vi "Serial Port Receive.vi"(8 "error in (no error)":errorcluster, 11 "Port handle in":refnum<k24>) -> (0 "error out":errorcluster, 2 "Message":u8[](array[numeric]) format="%.0x", 3 "Port handle out":refnum<k24>)   [LabVIEW 2015, in "VC940.lvlib"]
uses:
  VC940.lvlib
panel:
  out "Iteration":i32
  out "Message interval/ms":u32
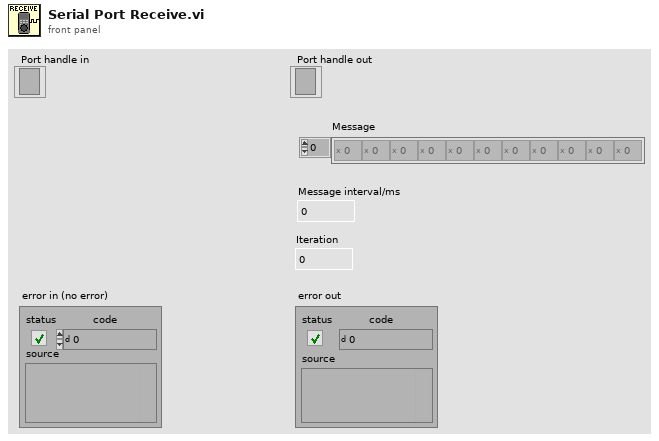
[diagram p1: front panel]
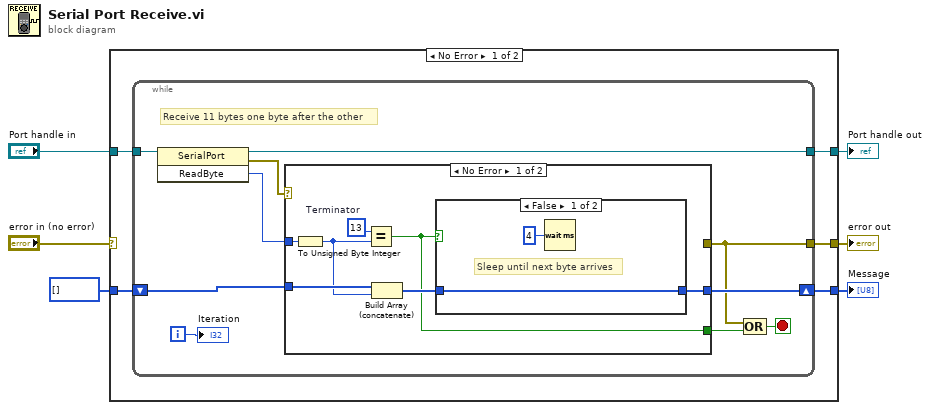
[diagram p0: block diagram]
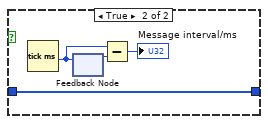
[diagram p2: hidden frame]
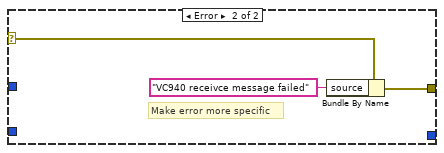
[diagram p3: hidden frame]
diagram:
  n1 = case shown="No Error" "error in (no error)" {
    selector: "error in (no error)" -> [_ w39]
    tunnel: [w11 w38] -> w6
    tunnel: "Port handle in" -> [w10 w38]
    tunnel: [w8 w39] -> w3
    tunnel: [w9 _] -> w2
    tunnel: u8[] [] ("appended array") -> [w7 _]
    frame No Error {
      n2 = while {
        tunnel: w10 -> [w21]
        tunnel: [w20] -> w11
        shift-right: [w16] -> w9
        shift-left: w7 -> [w17]
        tunnel: [w12] -> w8
        i -> [w19]
        stop <- w14 stop-if-true
        # "Receive 11 bytes one byte after the other"
        n3 = invoke class="SerialPort" method="ReadByte"(reference=w21) -> (reference out=w20:refnum<k24>, error out=w13:errorcluster, "ReadByte"=w18:i32)  [unwired: 2 in]
        n4 = case shown="No Error" w13 {
          selector: w13 -> [_ w37]
          tunnel: w18 -> [w28 _]
          tunnel: w17 -> [w27 _]
          tunnel: [w26 _] -> w16
          tunnel: [w24 _] -> w15
          tunnel: [_ w36] -> w12
          frame No Error {
            w22 = u8 13  # Terminator
            n5 = To Unsigned Byte Integer(number=w28) -> (unsigned 8bit integer=w23:u8)
            n6 = Equal?(x=w22, y=w23) -> (x = y?=w24:bool)
            n7 = Build Array (concatenate)(w27, w23) -> (w25:u8[])
            n8 = case shown="False" w24 {
              tunnel: w25 -> [w30 w31]
              tunnel: [w30 w31] -> w26
              frame False {
                # "Sleep until next byte arrives"
                n9 = Wait (ms)(milliseconds to wait=u32 4) -> ()  [unwired: 1 out]
              }
              frame True {
                n10 = Tick Count (ms)() -> (millisecond timer value=w33:u32)
                n11 = feedback-in #1(w33) -> ()
                n12 = feedback #1() -> (w34:u32)  [unwired: 1 in]
                n13 = Subtract(x=w33, y=w34) -> (x-y=→"Message interval/ms":u32)
              }
            }
          }
          frame Error {
            # "Make error more specific"
            n14 = Bundle By Name(cluster=w37, "source"="VC940 receivce message failed") -> (w36:errorcluster)
          }
        }
        n15 = Compound Arithmetic op=OR(w12, w15) -> (w14:bool)
        "Iteration" <- w19
      }
    }
    frame Error {
    }
  }
  "Port handle out" <- w6
  "error out" <- w3
  "Message" <- w2
